vi "Tester.vi"() -> ()   [LabVIEW 2021, in "EventSourceActor.lvlib" / "Event Source.lvlib" / "Event Source Actor.lvclass"]
uses:
  Event Source Actor.lvclass
  Event Source Actor.lvclass/Event Source Actor.ctl
  <vilib>/ActorFramework/Message Queue/Message Queue.lvclass
  <vilib>/ActorFramework/Message Dequeuer/Message Dequeuer.lvclass
  Event Data/Event Data.lvclass
panel:
  out "Msg":string
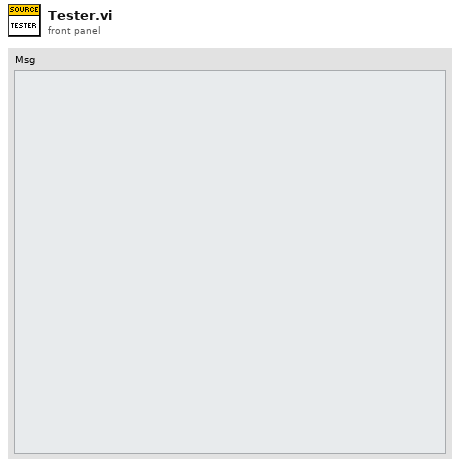
[diagram p1: front panel]
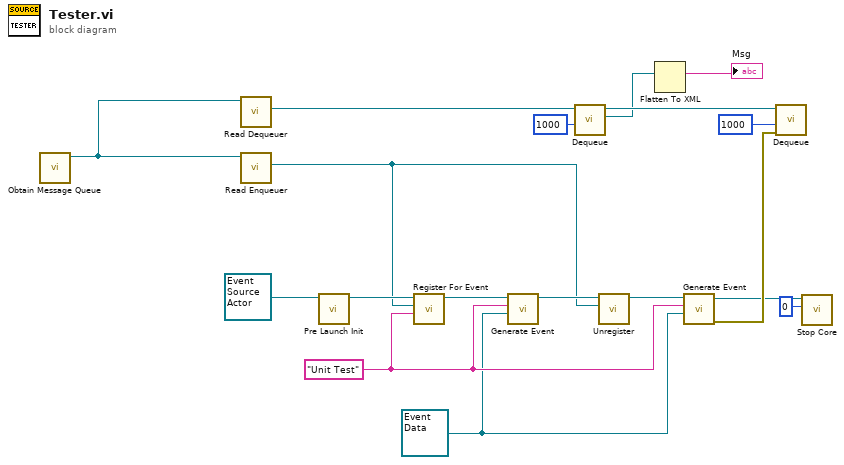
[diagram p0: block diagram]
diagram:
  w4 = refnum<class "Event Data.lvclass"> refnum ("Event Data")
  w5 = "Unit Test" ("Event Name")
  n1 = call <vilib>:"Obtain Message Queue.vi"() -> ("Message Queue"=w18:refnum<class "Message Queue.lvclass">)  [unwired: 10 in, 1 out]
  n2 = call <vilib>:"Read Dequeuer.vi"("Message Queue"=w18) -> ("Message Dequeuer"=w17:refnum<class "Message Dequeuer.lvclass">)  [unwired: 10 in]
  n3 = call <vilib>:"Read Enqueuer.vi"("Message Queue"=w18) -> ("Message Enqueuer"=w1:refnum<class "Message Enqueuer.lvclass">)  [unwired: 10 in]
  n4 = call-dynamic "Pre Launch Init.vi"("Event Source In"=refnum<class "Event Source Actor.lvclass"> refnum ("Event Source.lvlib:Event Source.lvclass")) -> ("Event Source Out"=w7:refnum<class "Event Source Actor.lvclass">)  [unwired: 9 in, 1 out]
  n5 = call-dynamic "Register For Event.vi"("Event Name"=w5, "Registrant Enq"=w1, "Event Source Actor In"=w7) -> ("Event Source Actor Out"=w6:refnum<class "Event Source Actor.lvclass">)  [unwired: 7 in, 1 out]
  n6 = call-dynamic "Generate Event.vi"("Event Data"=w4, "Event Name"=w5, "Event Source In"=w6) -> ("Event Source Out"=w8:refnum<class "Event Source Actor.lvclass">)  [unwired: 7 in, 1 out]
  n7 = call <vilib>:"Dequeue.vi"("timeout in ms (-1)"=1000, "Message Dequeuer in"=w17) -> ("Message"=w3:refnum<class "Message.lvclass">, "Message Dequeuer out"=w15:refnum<class "Message Dequeuer.lvclass">)  [unwired: 5 in, 3 out]
  n8 = call-dynamic "Unregister.vi"("Registrant Enq"=w1, "Event Source In"=w8) -> ("Event Source Out"=w16:refnum<class "Event Source Actor.lvclass">)  [unwired: 8 in, 1 out]
  n9 = Flatten To XML(6:w3) -> (2:→"Msg":string)
  n10 = call-dynamic "Generate Event.vi"("Event Data"=w4, "Event Name"=w5, "Event Source In"=w16) -> ("Error Out"=w13:errorcluster, "Event Source Out"=w11:refnum<class "Event Source Actor.lvclass">)  [unwired: 7 in]
  n11 = call <vilib>:"Dequeue.vi"("error in (no error)"=w13, "timeout in ms (-1)"=1000, "Message Dequeuer in"=w15) -> ()  [unwired: 4 in, 5 out]
  n12 = call-dynamic "Stop Core.vi"("final error code"=0, "Event Source In"=w11) -> ()  [unwired: 9 in, 1 out]
